vi "OnValueChange_rightUserTwo.vi"(8 "error in (no error)":errorcluster, 9 "Value":bool, 11 "Game in":refnum<class "Game.lvclass">) -> (0 "error out":errorcluster, 3 "Game out":refnum<class "Game.lvclass">)   [LabVIEW 2019, in "RT_Game.lvlib" / "Game.lvclass"]
uses:
  Game.lvclass
  Engine/ChangeVolumeData.ctl
  Engine/Engine.lvclass
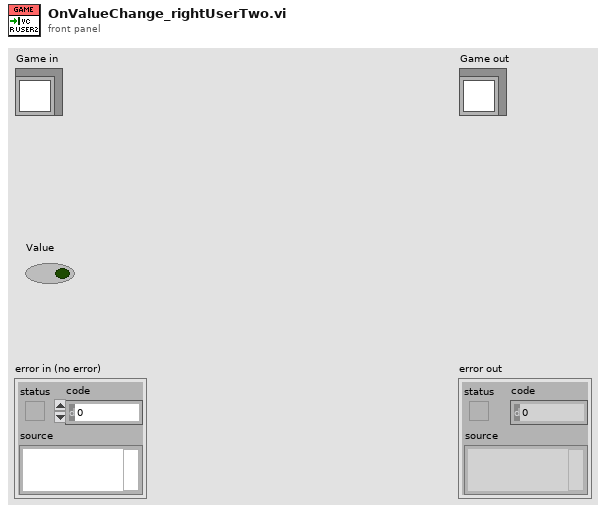
[diagram p1: front panel]
types:
  T1 = typedef "RT_Game.lvlib/Engine.lvclass/ChangeVolumeData.ctl" = enum16{"up", "down", "mute"}
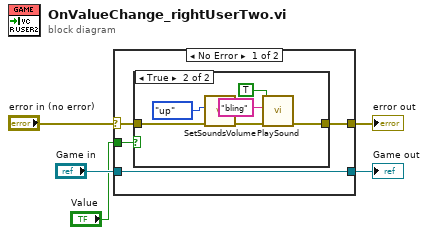
[diagram p0: block diagram]
diagram:
  n1 = case shown="No Error" "error in (no error)" {
    selector: "error in (no error)" -> [w8 w18]
    tunnel: [w7 w18] -> w4
    tunnel: [w9 w17] -> w2
    tunnel: "Game in" -> [w9 w17]
    tunnel: "Value" -> [w6 _]
    frame No Error {
      n2 = case shown="True" w6 {
        tunnel: w8 -> [w10 w16]
        tunnel: [w10 w13] -> w7
        frame False {
        }
        frame True {
          n3 = call "SetSoundsVolume.vi"("error in (no error)"=w16, "VolumeData"=ChangeVolumeData."up") -> ("error out"=w15:errorcluster)  [unwired: 9 in]
          n4 = call "PlaySound.vi"("error in (no error)"=w15, "Overwrite"=TRUE, "Name"="bling") -> ("error out"=w13:errorcluster)  [unwired: 8 in]
        }
      }
    }
    frame Error {
    }
  }
  "error out" <- w4
  "Game out" <- w2
